vi "Insert coverage as testcase.vi"(8 "Error in":errorcluster, 11 "Path instaCoverageReport":path caption="report path") -> (0 "error out":errorcluster)   [LabVIEW 2018]
uses:
  <vilib>/xml/Load XML File.vi
  <vilib>/xml/Close Reference(Node).vi
  <resource>/objmgr/DOMUserDefRef.rc
  <vilib>/xml/NI_XML.lvlib
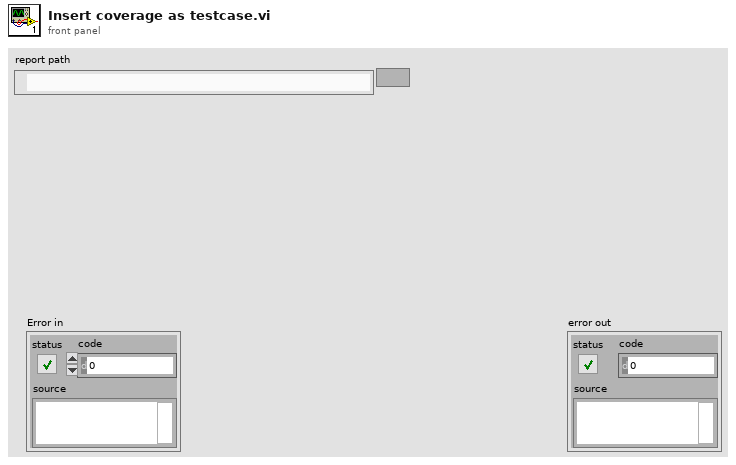
[diagram p1: front panel]
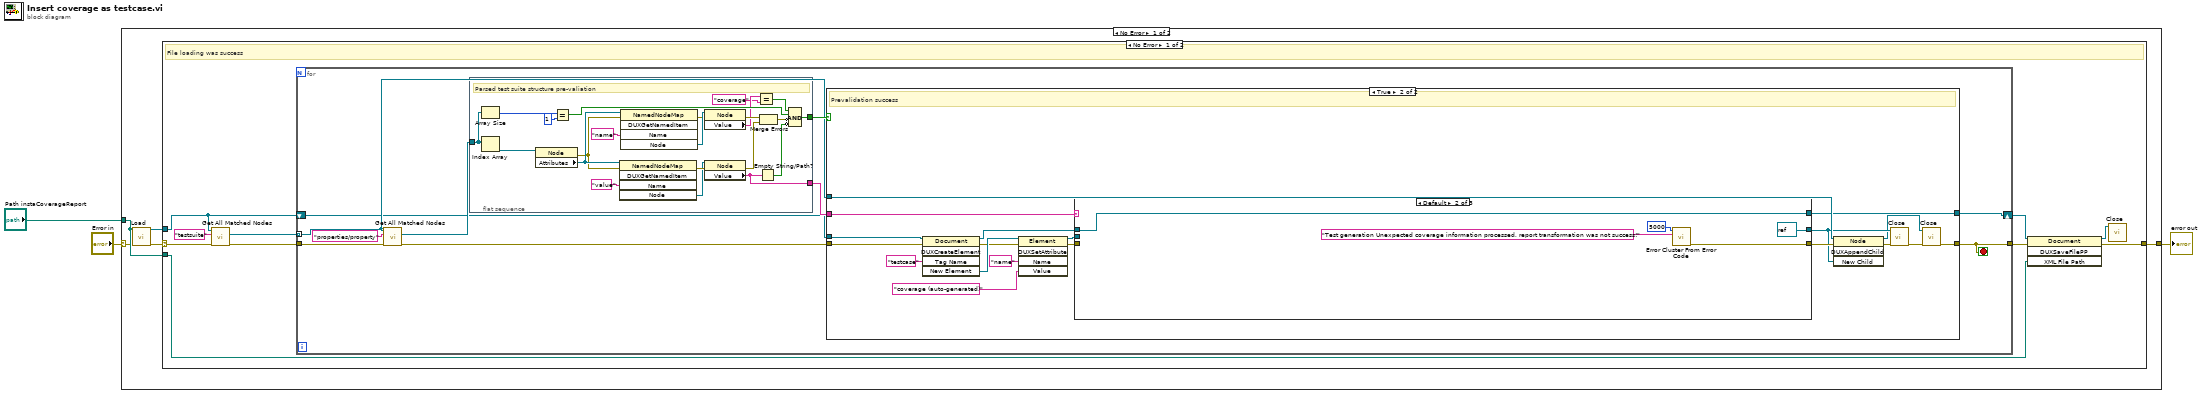
[diagram p0: block diagram]
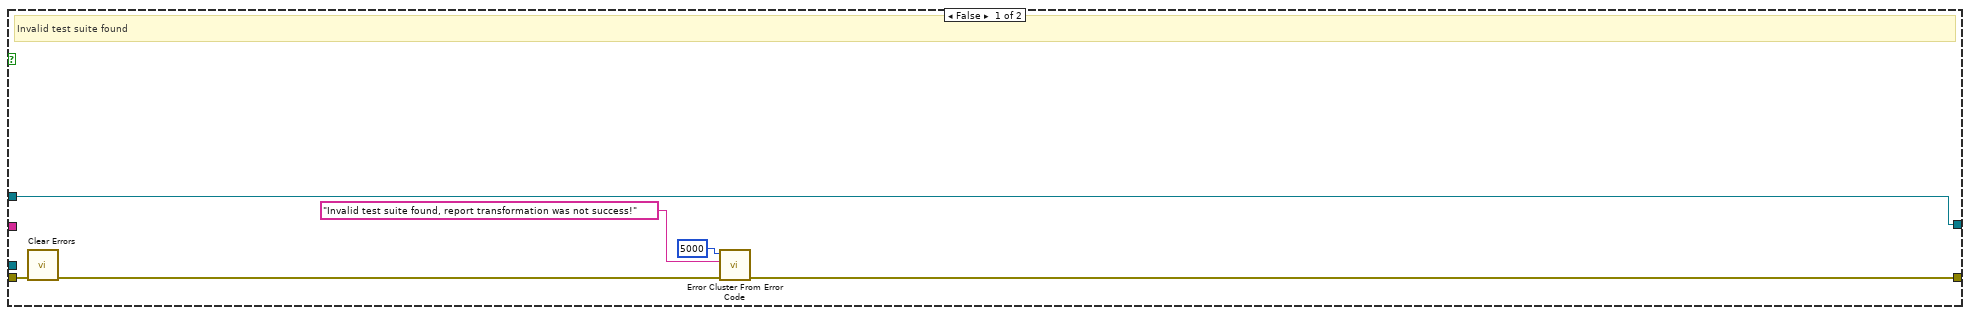
[diagram p2: hidden frame]
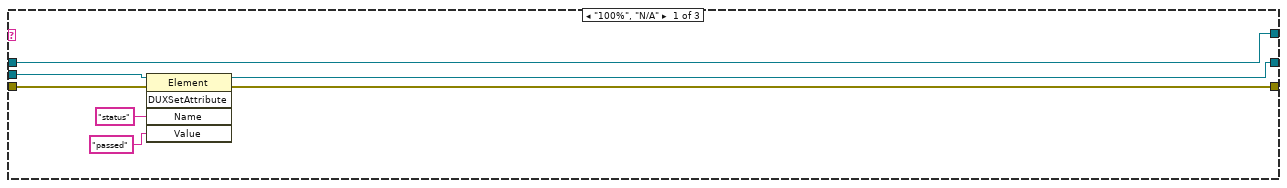
[diagram p3: hidden frame]
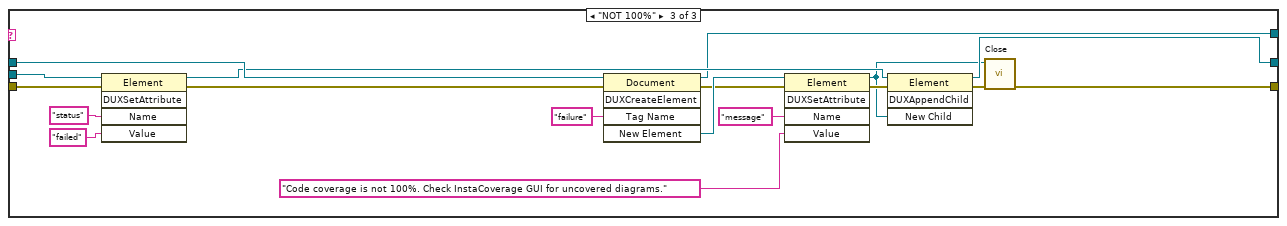
[diagram p4: hidden frame]
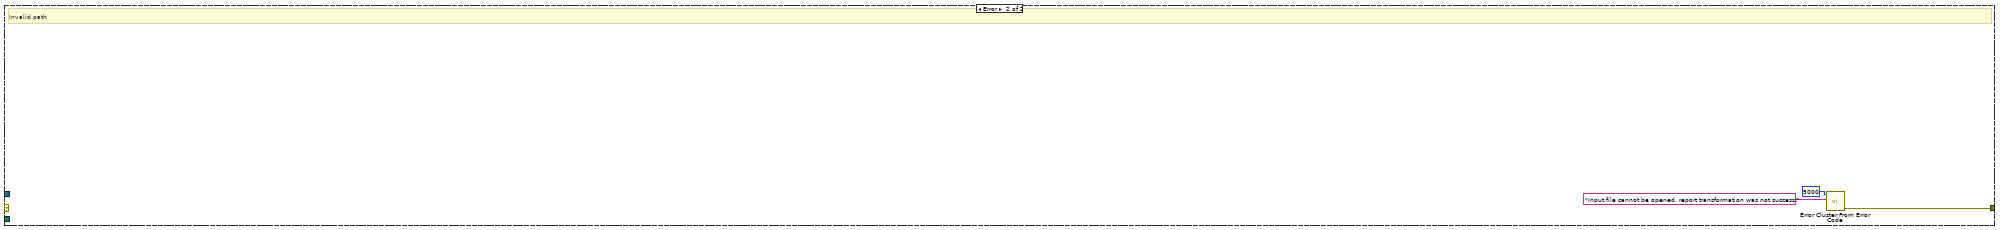
[diagram p5: hidden frame]
diagram:
  n1 = case shown="No Error" "Error in" {
    selector: "Error in" -> [w5 w109]
    tunnel: "Path instaCoverageReport" -> [w7 _]
    tunnel: [w6 w109] -> w2
    frame No Error {
      n2 = call-poly <vilib>:"Load.vi"("path to XML document"=w7, "error in (no error)"=w5) -> ("DOM document out"=w8:refnum<k20>, "error out"=w4:errorcluster)  [unwired: 11 in, 1 out]
      n3 = case shown="No Error" w4 {
        selector: w4 -> [w12 _]
        tunnel: w8 -> [w11 _]
        tunnel: w7 -> [w14 _]
        tunnel: [w13 w106] -> w6
        frame No Error {
          # "File loading was success"
          n4 = call <vilib>:"Get All Matched Nodes.vi"("error in (no error)"=w12, "XPath expression"="testsuite", "node in"=w11) -> ("error out"=w15:errorcluster, "node result array"=w16:refnum<k20>[])  [unwired: 6 in, 1 out]
          n5 = for {
            tunnel: w16 -> [w24] mode=indexing
            tunnel: w15 -> [w27]
            tunnel: [w22] -> w18
            shift-right: [w19] -> w9
            shift-left: w11 -> [w20]
            stop <- w22 stop-if-true
            n6 = call <vilib>:"Get All Matched Nodes.vi"("error in (no error)"=w27, "XPath expression"="properties/property", "node in"=w24) -> ("error out"=w26:errorcluster, "node result array"=w23:refnum<k20>[])  [unwired: 6 in, 1 out]
            n7 = flat-sequence {
              tunnel: w23 -> [w47]
              tunnel: [w36] -> w25
              tunnel: [w29] -> w21
              frame #0 {
                # "Parsed test suite structure pre-valiation"
                n8 = Array Size(array=w47) -> (size(s)=w50:i32)
                n9 = Index Array "Index Array"(array=w47) -> (element=w43:refnum<k20>)  [unwired: 1 in]
                n10 = property class="Node"(reference=w43) -> (error out=w34:errorcluster, "Attributes"=w35:refnum<k20>)  [unwired: 1 in, 1 out]
                n11 = Equal?(x=w50, y=1) -> (x = y?=w48:bool)
                n12 = invoke class="NamedNodeMap" method="DUXGetNamedItem"(reference=w35, error in=w34, "Name"="value") -> (error out=w42:errorcluster, "Node"=w41:refnum<k20>)  [unwired: 2 in, 3 out]
                n13 = invoke class="NamedNodeMap" method="DUXGetNamedItem"(reference=w35, error in=w34, "Name"="name") -> (error out=w44:errorcluster, "Node"=w45:refnum<k20>)  [unwired: 2 in, 3 out]
                n14 = property class="Node"(reference=w45, error in=w44) -> (error out=w39:errorcluster, "Value"=w33:string)  [unwired: 1 out]
                n15 = property class="Node"(reference=w41, error in=w42) -> (error out=w38:errorcluster, "Value"=w29:string)  [unwired: 1 out]
                n16 = Equal?(x=w33, y="coverage") -> (x = y?=w31:bool)
                n17 = Empty String/Path?(string/path=w29) -> (empty?=w30:bool)
                n18 = Merge Errors(w39, w38) -> (w37:errorcluster)
                n19 = Compound Arithmetic op=AND(w31, w48, invert w37, invert w30) -> (w36:bool)
              }
            }
            n20 = case shown="True" w25 {
              tunnel: w24 -> [w51 w75]
              tunnel: w20 -> [_ w74]
              tunnel: w26 -> [w53 w73]
              tunnel: [w56 w72] -> w22
              tunnel: w21 -> [_ w58]
              tunnel: [w51 w57] -> w19
              frame False {
                # "Invalid test suite found"
                n21 = call <vilib>:"Clear Errors.vi"("error in (no error)"=w53) -> ("error out"=w52:errorcluster)  [unwired: 5 in, 1 out]
                n22 = call <vilib>:"Error Cluster From Error Code.vi"("error in (no error)"=w52, "error message (\"\")"="Invalid test suite found, report transformation was not success!" ("error message (\"\")"), "error code (0)"=5000) -> ("error out"=w56:errorcluster)  [unwired: 6 in]
              }
              frame True {
                # "Prevalidation success"
                n23 = invoke class="Document" method="DUXCreateElement"(reference=w74, error in=w73, "Tag Name"="testcase") -> (reference out=w63:refnum<k20>, error out=w69:errorcluster, "New Element"=w70:refnum<k20>)  [unwired: 2 in, 2 out]
                n24 = invoke class="Element" method="DUXSetAttribute"(reference=w70, error in=w69, "Name"="name" ("Value"), "Value"="coverage (auto-generated)" ("Name")) -> (reference out=w66:refnum<k20>, error out=w65:errorcluster)  [unwired: 1 in, 3 out]
                n25 = case shown="Default" w58 {
                  tunnel: w66 -> [w82 _ w102]
                  tunnel: [w81 refnum<k20> refnum ("New Element") w92] -> w61
                  tunnel: w65 -> [w80 _ w103]
                  tunnel: [w79 w86 w89] -> w64
                  tunnel: w63 -> [w76 w83 w100]
                  tunnel: [w76 w83 w88] -> w57
                  frame "100%", "N/A" {
                    n26 = invoke class="Element" method="DUXSetAttribute"(reference=w82, error in=w80, "Name"="status", "Value"="passed") -> (reference out=w81:refnum<k20>, error out=w79:errorcluster)  [unwired: 1 in, 3 out]
                  }
                  frame Default {
                    n27 = call <vilib>:"Error Cluster From Error Code.vi"("error message (\"\")"="Test generation Unexpected coverage information processed, report transformation was not success!" ("error message (\"\")"), "error code (0)"=5000) -> ("error out"=w86:errorcluster)  [unwired: 7 in]
                  }
                  frame "NOT 100%" {
                    n28 = invoke class="Element" method="DUXSetAttribute"(reference=w102, error in=w103, "Name"="status", "Value"="failed") -> (reference out=w93:refnum<k20>, error out=w101:errorcluster)  [unwired: 1 in, 3 out]
                    n29 = invoke class="Document" method="DUXCreateElement"(reference=w100, error in=w101, "Tag Name"="failure") -> (reference out=w88:refnum<k20>, error out=w97:errorcluster, "New Element"=w98:refnum<k20>)  [unwired: 2 in, 2 out]
                    n30 = invoke class="Element" method="DUXSetAttribute"(reference=w98, error in=w97, "Name"="message", "Value"="Code coverage is not 100%. Check InstaCoverage GUI for uncovered diagrams.") -> (reference out=w91:refnum<k20>, error out=w94:errorcluster)  [unwired: 1 in, 3 out]
                    n31 = invoke class="Element" method="DUXAppendChild"(reference=w93, error in=w94, "New Child"=w91) -> (reference out=w92:refnum<k20>, error out=w90:errorcluster)  [unwired: 1 in, 2 out]
                    n32 = call-poly <vilib>:"Close.vi"("error in (no error)"=w90, "node"=w91) -> ("error out"=w89:errorcluster)  [unwired: 7 in]
                  }
                }
                n33 = invoke class="Node" method="DUXAppendChild"(reference=w75, error in=w64, "New Child"=w61) -> (reference out=w59:refnum<k20>, error out=w62:errorcluster)  [unwired: 1 in, 2 out]
                n34 = call-poly <vilib>:"Close.vi"("error in (no error)"=w62, "node"=w61) -> ("error out"=w60:errorcluster)  [unwired: 7 in]
                n35 = call-poly <vilib>:"Close.vi"("error in (no error)"=w60, "node"=w59) -> ("error out"=w72:errorcluster)  [unwired: 7 in]
              }
            }
          }
          n36 = invoke class="Document" method="DUXSaveFilePP"(reference=w9, error in=w18, "XML File Path"=w14) -> (reference out=w10:refnum<k20>, error out=w13:errorcluster)  [unwired: 1 in, 2 out]
          n37 = call-poly <vilib>:"Close.vi"("node"=w10) -> ()  [unwired: 8 in, 1 out]
        }
        frame Error {
          # "Invalid path"
          n38 = call <vilib>:"Error Cluster From Error Code.vi"("error message (\"\")"="Input file cannot be opened, report transformation was not success!" ("error message (\"\")"), "error code (0)"=5000) -> ("error out"=w106:errorcluster)  [unwired: 7 in]
        }
      }
    }
    frame Error {
    }
  }
  "error out" <- w2
